vi "Close UDV Refs.vi"(1 "UDVs in":T1[](array[typedef]) {"VS ref" format="%.0x"}) -> (0 "UDVs out":T1[](array[typedef]) {"VS ref" format="%.0x"})   [LabVIEW 2016, in "Scan Engine Custom Device.lvlib"]
uses:
  Scan Engine Custom Device.lvlib
  Type Defs/UDV Data.ctl
  <vilib>/NI Veristand/Custom Device API/Custom Device Item Ref.ctl
  Type Defs/UDV Data Type.ctl
  Type Defs/FXP Config.ctl
  <vilib>/NI Veristand/Custom Device API/Custom Device API.lvlib
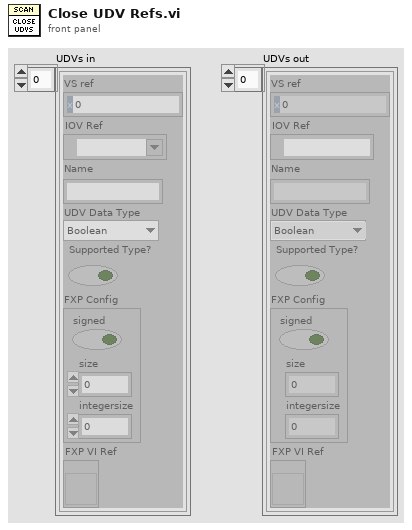
[diagram p1: front panel]
types:
  T1 = typedef "Scan Engine Custom Device.lvlib/UDV Data.ctl" = cluster{"VS ref":T2, "IOV Ref":refnum<k21>, "Name":string, "UDV Data Type":T3, "Supported Type?":bool, "FXP Config":T4, "FXP VI Ref":refnum<vi>}
  T2 = typedef "Custom Device API.lvlib/Custom Device Item Ref.ctl" = u64
  T3 = typedef "Scan Engine Custom Device.lvlib/UDV Data Type.ctl" = enum16{"Boolean", "Fixed Point", "Int8", "Int16", "Int32", "Int64", "U32 Bit Field", "UInt8", "UInt16", "UInt32", "UInt64", "Other"}
  T4 = typedef "Scan Engine Custom Device.lvlib/FXP Config.ctl" = cluster{"signed":bool, "size":u32, "integersize":i32}
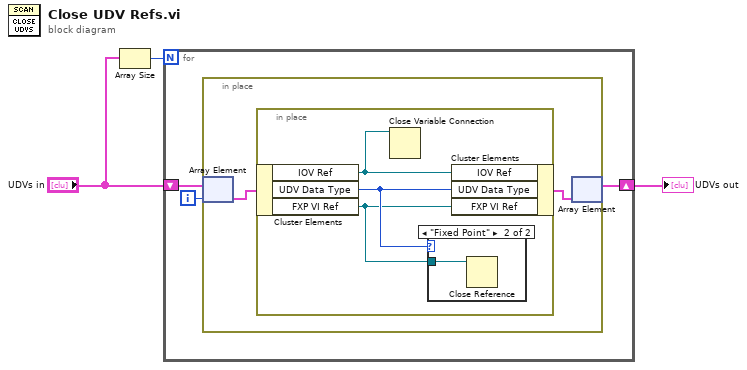
[diagram p0: block diagram]
diagram:
  n1 = Array Size(array="UDVs in") -> (size(s)=w1:i32)
  n2 = for {
    N: w1 -> [_]
    shift-right: [w5] -> w3
    shift-left: "UDVs in" -> [w6]
    i -> [w4]
    n3 = in-place {
      n4 = in-place-array #1(w6, w4) -> (w8:T1)
      n5 = in-place {
        n6 = in-place-cluster #2(w8) -> ("IOV Ref"=w9:refnum<k21>, "UDV Data Type"=w11:T3, "FXP VI Ref"=w10:refnum<vi>)
        n7 = Close Variable Connection(11:w9) -> ()  [unwired: 1 in, 1 out]
        n8 = case shown="\"Fixed Point\"" w11 {
          tunnel: w10 -> [_ w12]
          frame "Boolean", Default {
          }
          frame "Fixed Point" {
            n9 = Close Reference(reference=w12) -> ()  [unwired: 1 in, 1 out]
          }
        }
        n10 = in-place-cluster #2("IOV Ref"=w9, "UDV Data Type"=w11, "FXP VI Ref"=w10) -> (w7:T1)
      }
      n11 = in-place-array #1(w7) -> (w5:T1[])  [unwired: 1 out]
    }
  }
  "UDVs out" <- w3
